vi "Analog Logger.vi"() -> ()   [LabVIEW 2025]
panel:
  in  "Canal 3":string="Voltaje"
  in  "Canal 2":string="Porcentaje"
  in  "Canal 1":string="ADC"
  in  "Grupo":string="Analog read"
  in  "Cantidad de datos":i32
  out "Analog read":u16
  in  "Pin":u8=4 min=4 max=40
  out "error out":errorcluster
  in  "VISA resource name":refnum<visa-resource-name>
  in  "stop":bool
  # "Ejemplo: Lectura analógica y creación de reporte TDMS\nEste ejemplo muestra cómo adquirir una señal analógica y generar un reporte utilizando un VI personalizado que guarda los datos en formato TDMS en LV_ESP32.\nEntradas requeridas:\nPin_AI: Pin en el que se recibe la señal de voltaje analógico.\n\nParámetros del reporte: \nCantidad de datos, Grupo (Nombre de reporte), Canal 1, Canal 2, Canal 3\nRecibe 3 arreglos numericos que representan los datos de los canales antes mencionados  \n\nSalidas generadas:\nLectura analogica\nArchivo TDMS con los datos de la lectura analógica."
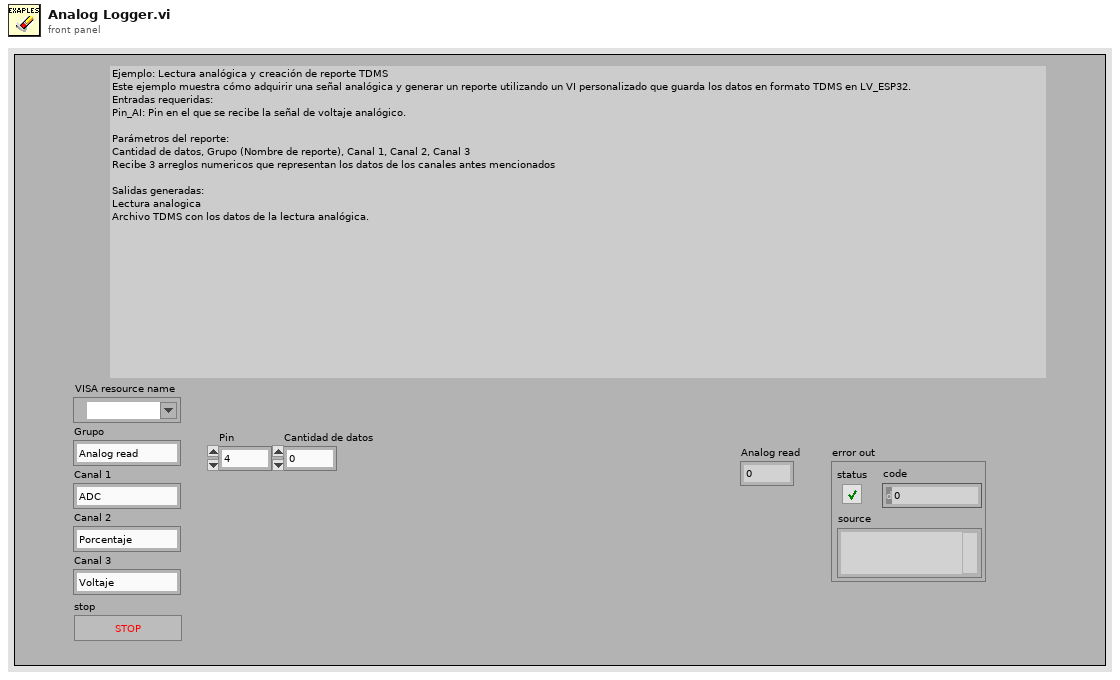
[diagram p1: front panel]
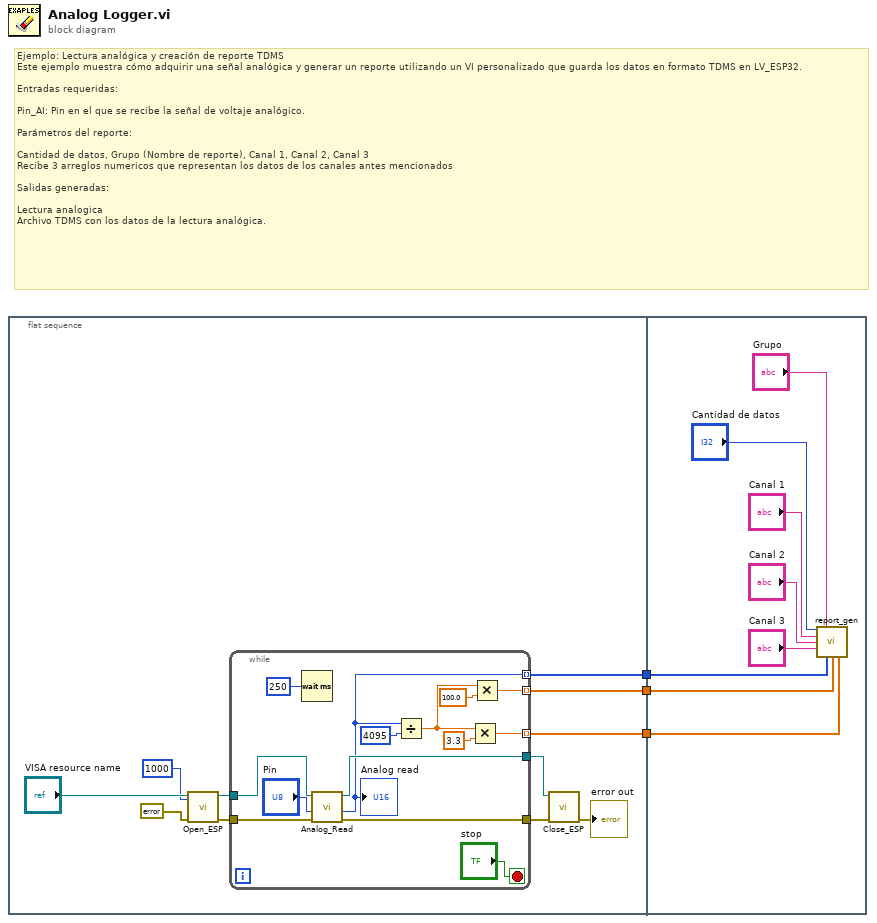
[diagram p0: block diagram]
diagram:
  # "Ejemplo: Lectura analógica y creación de reporte TDMS\nEste ejemplo muestra cómo adquirir una señal analógica y generar un reporte utilizando un VI personalizado que guarda los datos en formato TDMS en LV_ESP32.\n\nEntradas requeridas:\n\nPin_AI: Pin en el que se recibe la señal de voltaje analógico.\n\nParámetros del reporte: \n\nCantidad de datos, Grupo (Nombre de reporte), Canal 1, Canal 2, Canal 3\nRecibe 3 arreglos numericos que representan los datos de los canales antes mencionados  \n\nSalidas generadas:\n\nLectura analogica\nArchivo TDMS con los datos de la lectura analógica."
  n1 = flat-sequence {
    tunnel: [w6] -> w3
    tunnel: [w5] -> w2
    tunnel: [w4] -> w1
    tunnel: w3 -> [w31]
    tunnel: w2 -> [w30]
    tunnel: w1 -> [w29]
    frame #0 {
      n2 = call "Open_ESP.vi"("timeout (10sec)"=u32 1000, "error in (no error)"=errorcluster {"status"=FALSE, "code"=0, "source"=""}, "VISA resource name"="VISA resource name") -> ("error out"=w8:errorcluster, "VISA resource name out"=w14:refnum<visa-resource-name>)  [unwired: 7 in]
      n3 = while {
        tunnel: w14 -> [w27]
        tunnel: [w26] -> w11
        tunnel: [w25] -> w9
        tunnel: w8 -> [w24]
        tunnel: [w15] -> w6 mode=indexing
        tunnel: [w19] -> w5 mode=indexing
        tunnel: [w16] -> w4 mode=indexing
        stop <- "stop" stop-if-true
        n4 = Wait (ms)(milliseconds to wait=u32 250) -> ()  [unwired: 1 out]
        n5 = call "Analog_Read.vi"("error in (no error)"=w24, "Pin"="Pin", "VISA resource name"=w27) -> ("error out"=w25:errorcluster, "Analog read"=w15:u16, "VISA resource name out"=w26:refnum<visa-resource-name>)  [unwired: 6 in]
        "Analog read" <- w15
        n6 = Divide(x=w15, y=u16 4095) -> (x/y=w17:dbl)
        n7 = Multiply(x=w17, y=3.3) -> (x*y=w16:dbl)
        n8 = Multiply(x=w17, y=100.0) -> (x*y=w19:dbl)
      }
      n9 = call "Close_ESP.vi"("error in (no error)"=w9, "VISA resource name"=w11) -> ("error out"=→"error out":errorcluster)  [unwired: 9 in]
    }
    frame #1 {
      n10 = call "report_gen.vi"("Cantidad de datos"="Cantidad de datos", "Grupo"="Grupo", "Canal 1"="Canal 1", "Canal 2"="Canal 2", "Canal 3"="Canal 3", "Sensor 1"=w31, "Sensor 2"=w30, "Sensor 3"=w29) -> ()  [unwired: 7 in, 1 out]
    }
  }
